vi "Decode.vi"(8 "Error in":errorcluster, 11 "Encoded message":u8[](array[numeric]) format="%x") -> (0 "Error out":errorcluster, 3 "Decoded message":u8[](array[numeric]) format="%x")   [LabVIEW 2020, in "COBS.lvlib"]
uses:
  COBS.lvlib
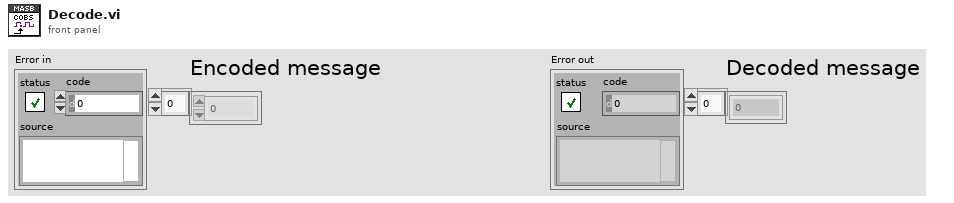
[diagram p1: front panel]
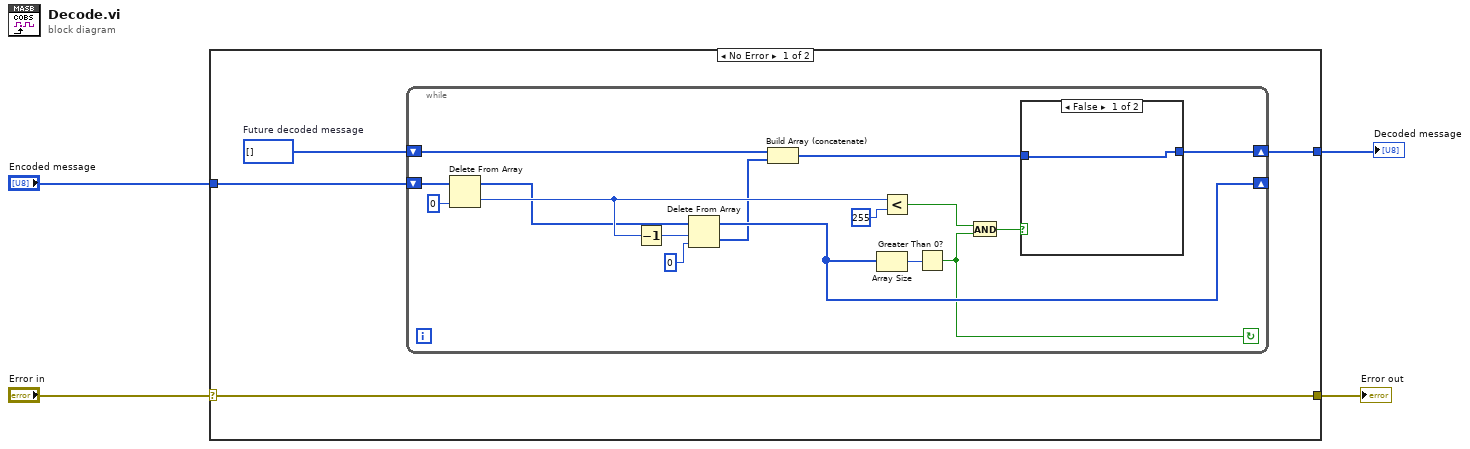
[diagram p0: block diagram]
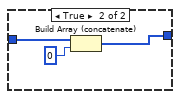
[diagram p2: hidden frame]
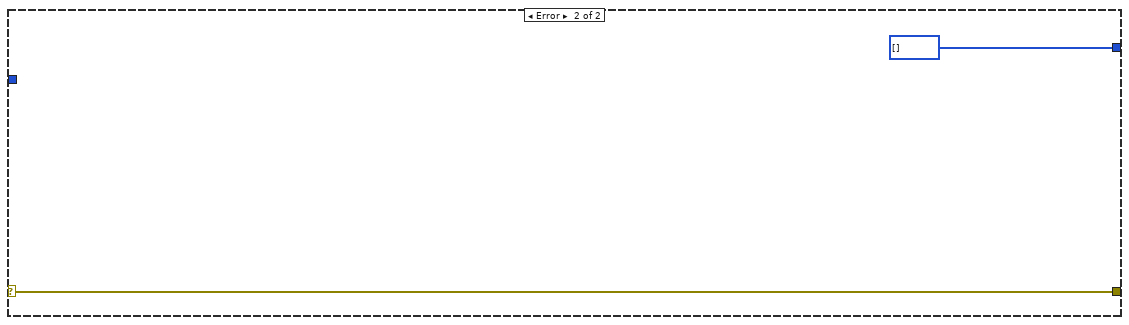
[diagram p3: hidden frame]
diagram:
  n1 = case shown="No Error" "Error in" {
    selector: "Error in" -> [w8 w30]
    tunnel: [w8 w30] -> w3
    tunnel: "Encoded message" -> [w7 _]
    tunnel: [w6 u8[] [] ("Future decoded message")] -> w1
    frame No Error {
      w5 = u8[] []  # Future decoded message
      n2 = while {
        shift-right: [w19] -> w6
        shift-left: w5 -> [w24]
        shift-right: [w18] -> _
        shift-left: w7 -> [w16]
        stop <- w17 continue-if-true
        n3 = Delete From Array(array=w16, index=0 ("length")) -> (deleted portion=w15:u8, array with subset deleted=w14:u8[])  [unwired: 1 in]
        n4 = Decrement(x=w15) -> (x-1=w10:u8)
        n5 = Delete From Array(array=w14, length=w10, index=0) -> (deleted portion=w13:u8[], array with subset deleted=w18:u8[])
        n6 = Build Array (concatenate)(w24, w13) -> (w20:u8[])
        n7 = Array Size(array=w18) -> (size(s)=w21:i32)
        n8 = Less?(x=w15, y=u8 255) -> (x < y?=w22:bool)
        n9 = Greater Than 0?(x=w21) -> (x > 0?=w17:bool)
        n10 = And(x=w22, y=w17) -> (x .and. y?=w9:bool)
        n11 = case shown="False" w9 {
          tunnel: w20 -> [w25 w28]
          tunnel: [w25 w26] -> w19
          frame False {
          }
          frame True {
            n12 = Build Array (concatenate)(w28, u8 0) -> (w26:u8[])
          }
        }
      }
    }
    frame Error {
    }
  }
  "Error out" <- w3
  "Decoded message" <- w1
